vi "用户登录.vi"() -> ()   [LabVIEW 2018]
panel:
  out "当前时间":timestamp format="%<%H:%M:%S >T"
  in  "选项卡控件":enum32{"主界面", "设置界面"}(tab)
  in  "时间":bool
  in  "退出登录":bool
  in  "用户名":string(combo)
  in  "设置密码":bool
  in  "注销按钮":bool
  in  "确定按钮":bool
  in  "密码":string
  in  "正确密码":string
  in  "返回主界面":bool
  in  "确认修改":bool
  in  "新密码":string="zxc"
  # "用户登录界面"
  # "修改密码界面"
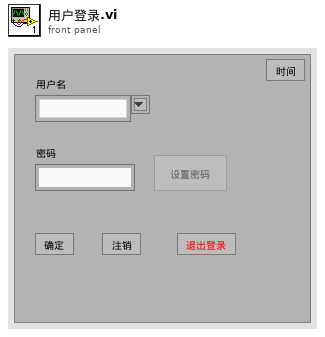
[diagram p1: front panel]
types:
  T1 = enum8{"Enabled", "Disabled", "Disabled and Grayed Out"}
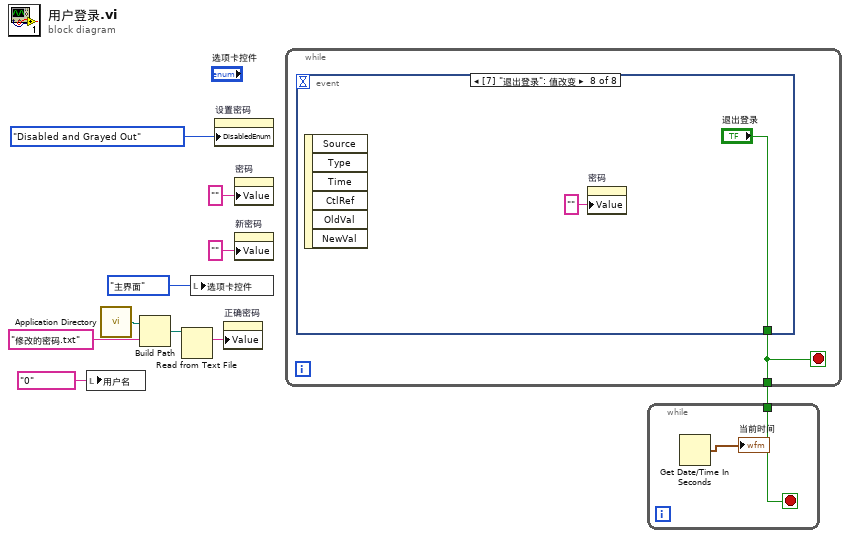
[diagram p0: block diagram]
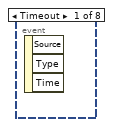
[diagram p2: hidden frame]
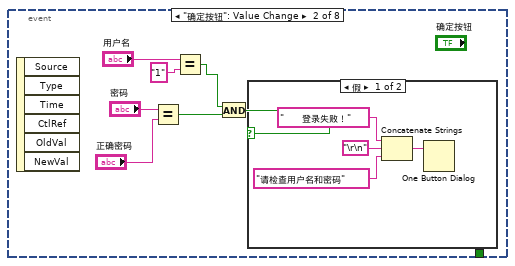
[diagram p3: hidden frame]
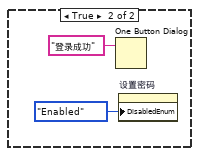
[diagram p4: hidden frame]
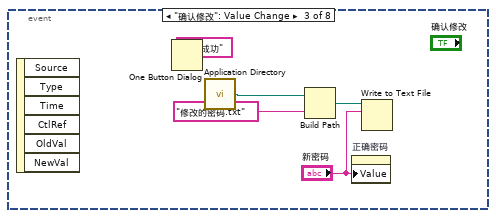
[diagram p5: hidden frame]
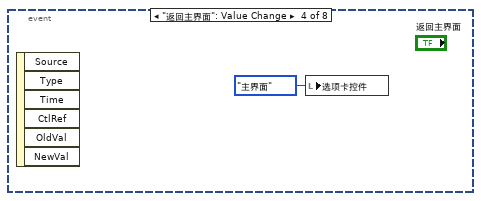
[diagram p6: hidden frame]
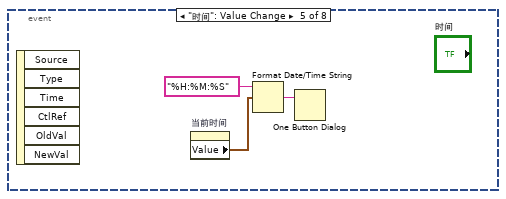
[diagram p7: hidden frame]
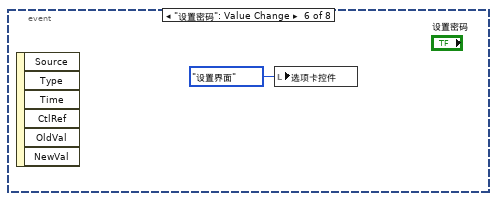
[diagram p8: hidden frame]
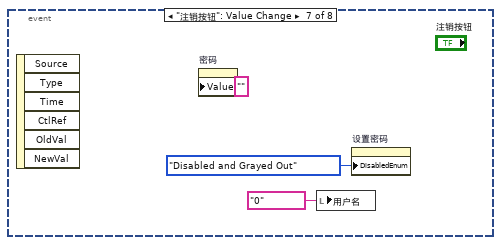
[diagram p9: hidden frame]
diagram:
  n1 = local write "用户名"("0" ("用户名")) -> ()
  n2 = call <vilib>:"Application Directory.vi"() -> ("Application Directory"=w5:path)
  n3 = Build Path(base path=w5, name or relative path="修改的密码.txt" ("名称或相对路径")) -> (appended path=w4:path)
  n4 = Read from Text File(file (use dialog)=w4) -> (text=w3:string)  [unwired: 3 in, 3 out]
  n5 = local write "选项卡控件"(enum32{"主界面", "设置界面"}."主界面" ("选项卡控件")) -> ()
  n6 = property on="设置密码" class="Bool"("DisabledEnum"=T1."Disabled and Grayed Out" ("禁用")) -> ()  [unwired: 2 in, 2 out]
  n7 = property on="正确密码" class="Str"("Value"=w3) -> ()  [unwired: 2 in, 2 out]
  n8 = property on="密码" class="Str"("Value"="" ("密码")) -> ()  [unwired: 2 in, 2 out]
  n9 = property on="新密码" class="Str"("Value"="" ("新密码")) -> ()  [unwired: 2 in, 2 out]
  n10 = while {
    tunnel: [w11] -> w1
    stop <- w11 stop-if-true
    n11 = event shown="[7] \"退出登录\": 值改变" {
      selector: _ -> [_ _ _ _ _ _ _ _]
      dyn-events: _ -> [_ _ _ _ _ _ _ _]
      timeout: _ -> [_ _ _ _ _ _ _ _]
      tunnel: [_ _ _ _ _ _ _ "退出登录"] -> w11
      event Timeout {
        n12 = event-data() -> ()  [unwired: 1 in, 3 out]
      }
      event "确定按钮": Value Change {
        n13 = event-data() -> ()  [unwired: 1 in, 6 out]
        n14 = Equal?(x="密码", y="正确密码") -> (x = y?=w13:bool)
        n15 = Equal?(x="用户名", y="1") -> (x = y?=w12:bool)
        n16 = And(x=w12, y=w13) -> (x .and. y?=w15:bool)
        n17 = case shown="假" w15 {
          frame False {
            n18 = Concatenate Strings("      登录失败！" ("字符串"), "\r\n", "请检查用户名和密码" ("字符串")) -> (w19:string)
            n19 = One Button Dialog(message=w19) -> ()  [unwired: 1 in, 1 out]
          }
          frame True {
            n20 = One Button Dialog(message="登录成功" ("消息")) -> ()  [unwired: 1 in, 1 out]
            n21 = property on="设置密码" class="Bool"("DisabledEnum"=T1."Enabled" ("禁用")) -> ()  [unwired: 2 in, 2 out]
          }
        }
      }
      event "确认修改": Value Change {
        n22 = event-data() -> ()  [unwired: 1 in, 6 out]
        n23 = One Button Dialog(message="修改成功" ("消息")) -> ()  [unwired: 1 in, 1 out]
        n24 = call <vilib>:"Application Directory.vi"() -> ("Application Directory"=w27:path)
        n25 = Build Path(base path=w27, name or relative path="修改的密码.txt" ("名称或相对路径")) -> (appended path=w28:path)
        n26 = property on="正确密码" class="Str"("Value"="新密码") -> ()  [unwired: 2 in, 2 out]
        n27 = Write to Text File(file (use dialog)=w28, text="新密码") -> ()  [unwired: 2 in, 3 out]
      }
      event "返回主界面": Value Change {
        n28 = event-data() -> ()  [unwired: 1 in, 6 out]
        n29 = local write "选项卡控件"(enum32{"主界面", "设置界面"}."主界面" ("选项卡控件")) -> ()
      }
      event "时间": Value Change {
        n30 = event-data() -> ()  [unwired: 1 in, 6 out]
        n31 = property on="当前时间" class="AbsTime (严格)"() -> ("Value"=w32:timestamp)  [unwired: 2 in, 2 out]
        n32 = Format Date/Time String(time format string (%c)="%H:%M:%S" ("时间格式字符串(%c)"), seconds (now)=w32) -> (date/time string=w31:string)  [unwired: 1 in]
        n33 = One Button Dialog(message=w31) -> ()  [unwired: 1 in, 1 out]
      }
      event "设置密码": Value Change {
        n34 = event-data() -> ()  [unwired: 1 in, 6 out]
        n35 = local write "选项卡控件"(enum32{"主界面", "设置界面"}."设置界面" ("选项卡控件")) -> ()
      }
      event "注销按钮": Value Change {
        n36 = event-data() -> ()  [unwired: 1 in, 6 out]
        n37 = property on="密码" class="Str"("Value"="" ("密码")) -> ()  [unwired: 2 in, 2 out]
        n38 = local write "用户名"("0" ("用户名")) -> ()
        n39 = property on="设置密码" class="Bool"("DisabledEnum"=T1."Disabled and Grayed Out" ("禁用")) -> ()  [unwired: 2 in, 2 out]
      }
      event "退出登录": Value Change {
        n40 = event-data() -> ()  [unwired: 1 in, 6 out]
        n41 = property on="密码" class="Str"("Value"="" ("密码")) -> ()  [unwired: 2 in, 2 out]
      }
    }
  }
  n42 = while {
    tunnel: w1 -> [w40]
    stop <- w40 stop-if-true
    n43 = Get Date/Time In Seconds() -> (seconds since 1Jan1904=→"当前时间":timestamp)
  }
